vi "niRFSTS RFPM Initialize.vi"(11 "TSM Context":T1) -> (0 "error out":errorcluster)   [LabVIEW 2014]
uses:
  <vilib>/NI_TestStand_SemiconductorModule/NI_TestStand_Semiconductor_Module.lvlibp/PinMap/General/SemiconductorModuleContext.ctl
  <vilib>/NI_TestStand_SemiconductorModule/NI_TestStand_Semiconductor_Module.lvlibp
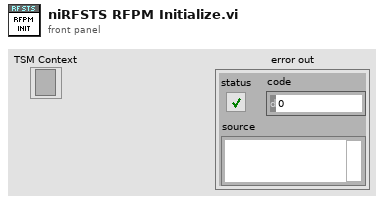
[diagram p1: front panel]
types:
  T1 = typedef "NI_TestStand_Semiconductor_Module.lvlibp/SemiconductorModuleContext.ctl" = refnum<k7>
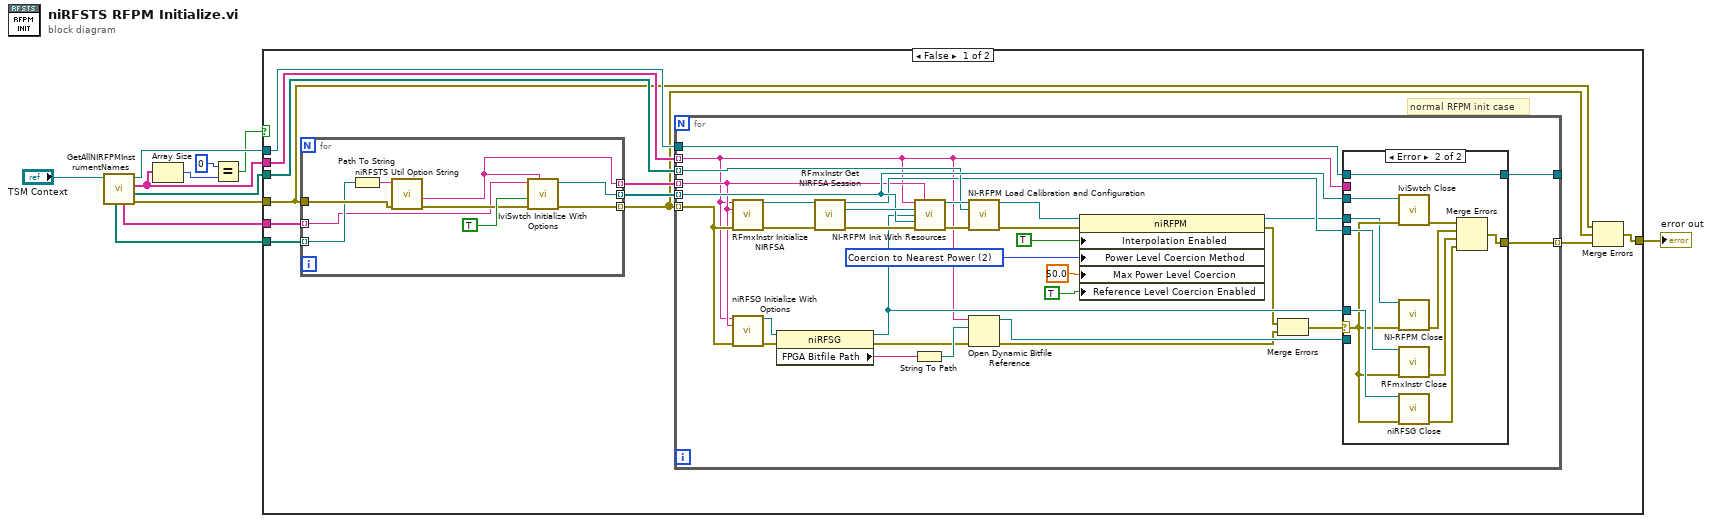
[diagram p0: block diagram]
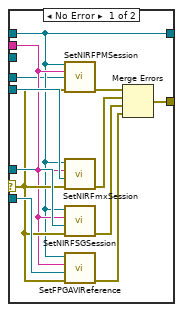
[diagram p2: hidden frame]
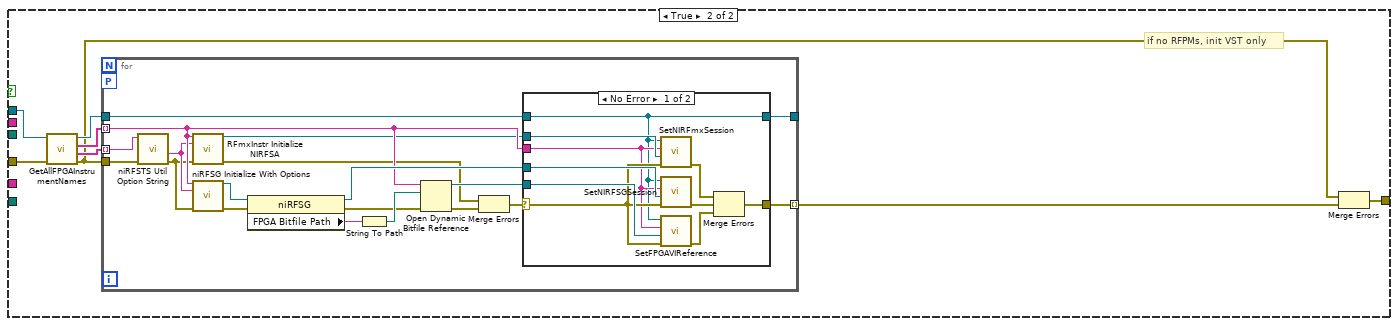
[diagram p3: hidden frame]
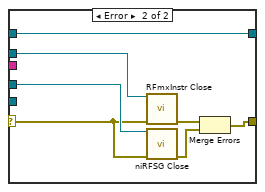
[diagram p4: hidden frame]
diagram:
  n1 = call <vilib>:"GetAllNIRFPMInstrumentNames.vi"("Semiconductor Module Context"="TSM Context") -> ("error out"=w7:errorcluster, "Calibration File Paths"=w11:path[], "Instrument Names"=w6:string[], "Semiconductor Module Context out"=w9:T1, "IVI Switch Names"=w8:string[], "FPGA File Paths"=w10:path[])  [unwired: 5 in]
  n2 = Array Size(array=w6) -> (size(s)=w5:i32)
  n3 = Equal?(x=0, y=w5) -> (x = y?=w3:bool)
  n4 = case shown="False" w3 {
    tunnel: [w12 w88] -> w1
    tunnel: w11 -> [w19 _]
    tunnel: w10 -> [w18 _]
    tunnel: w9 -> [w17 w93]
    tunnel: w8 -> [w16 _]
    tunnel: w7 -> [w13 w94]
    tunnel: w6 -> [w15 _]
    frame False {
      # "normal RFPM init case"
      n5 = for {
        tunnel: [w26] -> w21 mode=indexing
        tunnel: [w29] -> w14 mode=indexing
        tunnel: w13 -> [w28]
        tunnel: [w27] -> w20 mode=indexing
        tunnel: w16 -> [w23] mode=indexing
        tunnel: w18 -> [w25] mode=indexing
        n6 = Path To String(path=w25) -> (string=w24:string)
        n7 = call "niRFSTS Util Option String.vi"("error in (no error)"=w28, "FPGA File Path"=w24) -> ("error out"=w30:errorcluster, "FPGA Option String"=w26:string)  [unwired: 6 in, 2 out]
        n8 = call <vilib>:"IviSwtch Initialize With Options.vi"("option string (\"Simulate=0,RangeCheck=1,QueryInstrStatus=0,Cache=1\")"=w26, "error in (no error)"=w30, "reset device (True)"=TRUE ("reset"), "logical name (\"SampleSwitch\")"=w23) -> ("error out"=w29:errorcluster, "instrument handle out"=w27:refnum<k15>)  [unwired: 6 in]
      }
      n9 = for {
        tunnel: [w63] -> w22 mode=indexing
        tunnel: w21 -> [w44] mode=indexing
        tunnel: w14 -> [w46] mode=indexing
        tunnel: w20 -> [w58] mode=indexing
        tunnel: w15 -> [w41] mode=indexing
        tunnel: w19 -> [w57] mode=indexing
        tunnel: w17 -> [w56]
        tunnel: [w40] -> _
        w37 = 2 items=["Coercion Disabled"=1, "Coercion to Nearest Power"=2, "Coercion to Lower Power"=3] ("Measurement:Power Level Coercion Method")
        n10 = call <vilib>:"RFmxInstr Initialize NIRFSA.vi"("Resource Name"=w41, "Option String"=w44, "error in (no error)"=w46) -> ("Instrument Handle Out"=w54:refnum<k21>, "error out"=w55:errorcluster)  [unwired: 10 in, 1 out]
        n11 = call <instrlib>:"niRFSG Initialize With Options.vi"("resource name"=w41, "option string"=w44, "error in"=w46) -> ("instrument handle"=w52:refnum<k15>, "error out"=w50:errorcluster)  [unwired: 11 in]
        n12 = property class="niRFSG"(reference=w52, error in=w50) -> (reference out=w47:refnum<k15>, error out=w49:errorcluster, "FPGA Bitfile Path"=w51:string)
        n13 = call <vilib>:"RFmxInstr Get NIRFSA Session.vi"("Instrument Handle In"=w54, "error in (no error)"=w55) -> ("Instrument Handle Out"=w48:refnum<k21>, "NI RFSA Session"=w61:refnum<k15>, "error out"=w62:errorcluster)  [unwired: 11 in]
        n14 = String To Path(string=w51) -> (path=w53:path)
        n15 = call <instrlib>:"NI-RFPM Init With Resources.vi"("resource name"=w41, "option string"=w44, "RFSA handle"=w61, "RFSG handle"=w47, "Switch handle"=w58, "error in"=w62) -> ("instrument handle out"=w59:refnum<k15>, "error out"=w60:errorcluster)  [unwired: 8 in]
        n16 = call <instrlib>:"NI-RFPM Load Calibration and Configuration.vi"("NI-5530 handle in"=w59, "Calibration Storage File Path"=w57, "error in"=w60) -> ("instrument handle out"=w39:refnum<k15>, "error out"=w33:errorcluster)  [unwired: 11 in]
        n17 = Open Dynamic Bitfile Reference(0:w41, 1:w53, 3:w49) -> (5:w45:refnum<k20>, 8:w42:errorcluster)  [unwired: 2 in]
        n18 = property class="niRFPM"(reference=w39, error in=w33, "Interpolation Enabled"=TRUE ("Measurement:Interpolation Enabled"), "Power Level Coercion Method"=w37, "Max Power Level Coercion"=50.0 ("Measurement:Maximum Power Level Coercion"), "Reference Level Coercion Enabled"=TRUE ("Measurement:Reference Level Coercion Enabled")) -> (reference out=w34:refnum<k15>, error out=w32:errorcluster)
        n19 = Merge Errors(w32, w42) -> (w43:errorcluster)
        n20 = case shown="Error" w43 {
          selector: w43 -> [w68 w80]
          tunnel: [w70 w85] -> w63
          tunnel: w58 -> [_ w84]
          tunnel: w56 -> [w65 w77]
          tunnel: w48 -> [w75 w81]
          tunnel: w47 -> [w74 w82]
          tunnel: w45 -> [w69 _]
          tunnel: w41 -> [w66 _]
          tunnel: [w65 w77] -> w40
          tunnel: w34 -> [w64 w76]
          frame No Error {
            n21 = call <vilib>:"SetNIRFPMSession.vi"("Semiconductor Module Context"=w65, "Instrument Name"=w66, "NI-RFPM Session"=w64, "error in (no error)"=w68) -> ("error out"=w73:errorcluster)  [unwired: 10 in, 1 out]
            n22 = call <vilib>:"SetNIRFmxSession.vi"("error in (no error)"=w68, "NI-RFmx Session"=w75, "Instrument Name"=w66, "Semiconductor Module Context"=w65) -> ("error out"=w72:errorcluster)  [unwired: 6 in, 1 out]
            n23 = call <vilib>:"SetNIRFSGSession.vi"("error in (no error)"=w68, "NI-RFSG Session"=w74, "Instrument Name"=w66, "Semiconductor Module Context"=w65) -> ("error out"=w71:errorcluster)  [unwired: 6 in, 1 out]
            n24 = call <vilib>:"SetFPGAVIReference.vi"("error in (no error)"=w68, "FPGA VI Reference"=w69, "Instrument Name"=w66, "Semiconductor Module Context"=w65) -> ("error out"=w67:errorcluster)  [unwired: 6 in, 1 out]
            n25 = Merge Errors(w73, w72, w71, w67) -> (w70:errorcluster)
          }
          frame Error {
            n26 = call <vilib>:"IviSwtch Close.vi"("error in (no error)"=w80, "instrument handle"=w84) -> ("error out"=w86:errorcluster)  [unwired: 9 in]
            n27 = call <instrlib>:"NI-RFPM Close.vi"("NI-5530 handle in"=w76, "error in"=w80) -> ("error out"=w83:errorcluster)  [unwired: 13 in]
            n28 = call <vilib>:"RFmxInstr Close.vi"("Instrument Handle In"=w81, "error in (no error)"=w80) -> ("error out"=w79:errorcluster)  [unwired: 13 in]
            n29 = call <instrlib>:"niRFSG Close.vi"("instrument handle"=w82, "error in"=w80) -> ("error out"=w78:errorcluster)  [unwired: 13 in]
            n30 = Merge Errors(w86, w83, w79, w78) -> (w85:errorcluster)
          }
        }
      }
      n31 = Merge Errors(w13, w14, w22) -> (w12:errorcluster)
    }
    frame True {
      # "if no RFPMs, init VST only"
      n32 = call <vilib>:"GetAllFPGAInstrumentNames.vi"("error in (no error)"=w94, "Semiconductor Module Context"=w93) -> ("error out"=w87:errorcluster, "FPGA File Paths"=w90:string[], "Instrument Names"=w92:string[], "Semiconductor Module Context Out"=w91:T1)  [unwired: 6 in]
      n33 = for {
        tunnel: [w113] -> w89 mode=indexing
        tunnel: w87 -> [w100]
        tunnel: w92 -> [w102] mode=indexing
        tunnel: w91 -> [w112]
        workers-P: _ -> [_]
        tunnel: w90 -> [w98] mode=indexing
        tunnel: [w95] -> _
        n34 = call "niRFSTS Util Option String.vi"("error in (no error)"=w100, "FPGA File Path"=w98) -> ("error out"=w99:errorcluster, "FPGA Option String"=w101:string)  [unwired: 6 in, 2 out]
        n35 = call <vilib>:"RFmxInstr Initialize NIRFSA.vi"("Resource Name"=w102, "Option String"=w101, "error in (no error)"=w99) -> ("Instrument Handle Out"=w97:refnum<k21>, "error out"=w96:errorcluster)  [unwired: 10 in, 1 out]
        n36 = call <instrlib>:"niRFSG Initialize With Options.vi"("resource name"=w102, "option string"=w101, "error in"=w99) -> ("instrument handle"=w110:refnum<k15>, "error out"=w108:errorcluster)  [unwired: 11 in]
        n37 = property class="niRFSG"(reference=w110, error in=w108) -> (reference out=w106:refnum<k15>, error out=w107:errorcluster, "FPGA Bitfile Path"=w109:string)
        n38 = String To Path(string=w109) -> (path=w111:path)
        n39 = Open Dynamic Bitfile Reference(0:w102, 1:w111, 3:w107) -> (5:w105:refnum<k20>, 8:w103:errorcluster)  [unwired: 2 in]
        n40 = Merge Errors(w96, w103) -> (w104:errorcluster)
        n41 = case shown="No Error" w104 {
          selector: w104 -> [w117 w127]
          tunnel: [w119 w130] -> w113
          tunnel: w112 -> [w114 w124]
          tunnel: w97 -> [w123 w128]
          tunnel: w106 -> [w122 w129]
          tunnel: w105 -> [w118 _]
          tunnel: w102 -> [w115 _]
          tunnel: [w114 w124] -> w95
          frame No Error {
            n42 = call <vilib>:"SetNIRFmxSession.vi"("error in (no error)"=w117, "NI-RFmx Session"=w123, "Instrument Name"=w115, "Semiconductor Module Context"=w114) -> ("error out"=w121:errorcluster)  [unwired: 6 in, 1 out]
            n43 = call <vilib>:"SetNIRFSGSession.vi"("error in (no error)"=w117, "NI-RFSG Session"=w122, "Instrument Name"=w115, "Semiconductor Module Context"=w114) -> ("error out"=w120:errorcluster)  [unwired: 6 in, 1 out]
            n44 = call <vilib>:"SetFPGAVIReference.vi"("error in (no error)"=w117, "FPGA VI Reference"=w118, "Instrument Name"=w115, "Semiconductor Module Context"=w114) -> ("error out"=w116:errorcluster)  [unwired: 6 in, 1 out]
            n45 = Merge Errors(w121, w120, w116) -> (w119:errorcluster)
          }
          frame Error {
            n46 = call <vilib>:"RFmxInstr Close.vi"("Instrument Handle In"=w128, "error in (no error)"=w127) -> ("error out"=w126:errorcluster)  [unwired: 13 in]
            n47 = call <instrlib>:"niRFSG Close.vi"("instrument handle"=w129, "error in"=w127) -> ("error out"=w125:errorcluster)  [unwired: 13 in]
            n48 = Merge Errors(w126, w125) -> (w130:errorcluster)
          }
        }
      }
      n49 = Merge Errors(w87, w89) -> (w88:errorcluster)
    }
  }
  "error out" <- w1
